vi "总氮总磷加标回收 (子VI).vi"   [LabVIEW 2016, in "质控单元.lvlib"]
types:
  T1 = cluster{"氨氮":bool, "总磷":bool, "总氮":bool, "CODMn":bool, "CODCr":bool}
  T2 = cluster{"是否启用仪器":bool, "CODMn":cluster{"启动测量模式":cluster{"测量模式":enum16{"水样测量", "标样核查", "加标回收", "平行样", "校零", "校标"}}, "确定按钮":bool}, "启动模块":cluster{"氨氮":bool, "总磷":bool, "总氮":bool, "COD":bool}, "常规启动":bool, "直接启动":bool}
  T3 = enum32{"Bad", "Idle", "Run top level", "Running"}
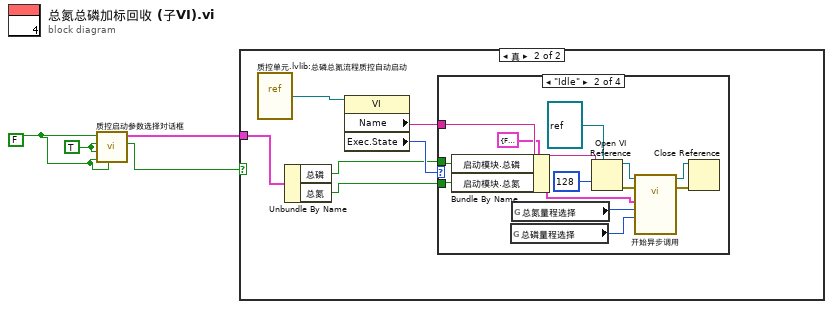
[diagram p0: block diagram]
diagram:
  w2 = TRUE ("总氮")
  w1 = FALSE ("氨氮")
  n1 = call "质控启动参数选择对话框.vi"("CODCr"=w1, "CODMn"=w1, "总氮"=w2, "总磷"=w2, "氨氮"=w1) -> ("确定启动"=w3:bool, "启动模块"=w4:T1)  [unwired: 4 in, 1 out]
  n2 = case shown="真" w3 {
    tunnel: w4 -> [_ w7]
    frame False {
    }
    frame True {
      n3 = vi-ref "质控单元.lvlib:总磷总氮流程质控自动启动.vi"() -> (w10:refnum<vi>)
      n4 = Unbundle By Name(w7) -> ("总磷"=w6:bool, "总氮"=w5:bool)
      n5 = property class="VI"(reference=w10) -> ("Name"=w8:string, "Exec.State"=w9:T3)  [unwired: 1 in, 2 out]
      n6 = case shown="\"Idle\"" w9 {
        tunnel: w8 -> [_ w19 _ _]
        tunnel: w6 -> [_ w14 _ _]
        tunnel: w5 -> [_ w13 _ _]
        frame "Bad", Default {
        }
        frame "Idle" {
          n7 = Bundle By Name(cluster=T2 {"是否启用仪器"=FALSE, "CODMn"={"启动测量模式"={"测量模式"=enum."水样测量"}, "确定按钮"=FALSE}, "启动模块"={"氨氮"=FALSE, "总磷"=FALSE, "总氮"=FALSE, "COD"=FALSE}, "常规启动"=FALSE, "直接启动"=FALSE} ("参数"), "启动模块.总磷"=w14, "启动模块.总氮"=w13) -> (w15:T2)
          n8 = global read "断电保存全局.vi" "总磷量程选择"() -> (w11:enum32{"H", "L", "AUTO"})
          n9 = global read "断电保存全局.vi" "总氮量程选择"() -> (w12:enum32{"H", "L", "AUTO"})
          n10 = Open VI Reference(type specifier VI Refnum (for type only)=refnum<vi> refnum ("类型说明符VI引用句柄（仅用于类型）"), vi path=w19, options=128 ("选项")) -> (vi reference=w23:refnum<vi>, error out=w17:errorcluster)  [unwired: 3 in]
          n11 = call-by-ref "开始异步调用"(reference=w23, error in=w17, "总磷量程切换"=w11, "总氮量程切换"=w12, "参数"=w15) -> (reference out=w22:refnum<vi>, error out=w18:errorcluster)  [unwired: 9 in]
          n12 = Close Reference(reference=w22, error in (no error)=w18) -> ()  [unwired: 1 out]
        }
        frame "Run top level" {
        }
        frame "Running" {
        }
      }
    }
  }
